vi "Interpolation Color.vi"(9 "Interpolation Value":dbl, 10 "Input Color2":u32(colorbox), 11 "Input Color1":u32(colorbox)) -> (3 "Output Color":u32(colorbox))   [LabVIEW 2020, in "3D Plot.lvclass"]
uses:
  <vilib>/Math Plots/3D Math Plots/3D Plot/3D Plot/3D Plot.lvclass
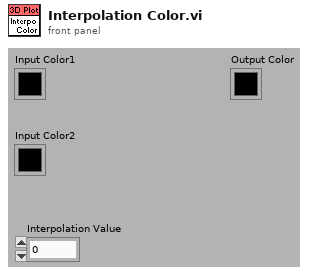
[diagram p1: front panel]
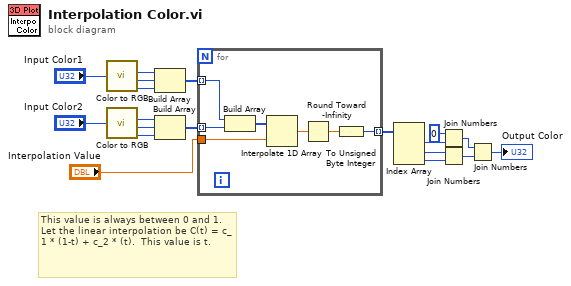
[diagram p0: block diagram]
diagram:
  # "This value is always between 0 and 1.  Let the linear interpolation be C(t) = c_1 * (1-t) + c_2 * (t).  This value is t."
  n1 = call <vilib>:"Color to RGB.vi"("Color"="Input Color1") -> ("R"=w1:u8, "G"=w2:u8, "B"=w3:u8)  [unwired: 1 out]
  n2 = call <vilib>:"Color to RGB.vi"("Color"="Input Color2") -> ("R"=w6:u8, "G"=w5:u8, "B"=w4:u8)  [unwired: 1 out]
  n3 = Build Array(w1, w2, w3) -> (w18:u8[])
  n4 = Build Array(w6, w5, w4) -> (w17:u8[])
  n5 = for {
    tunnel: w18 -> [w26] mode=indexing
    tunnel: w17 -> [w25] mode=indexing
    tunnel: "Interpolation Value" -> [w23]
    tunnel: [w20] -> w16 mode=indexing
    n6 = Build Array(w26, w25) -> (w24:u8[])
    n7 = Interpolate 1D Array(1:w23, 2:w24) -> (0:w22:dbl)
    n8 = Round Toward -Infinity(1:w22) -> (0:w21:dbl)
    n9 = To Unsigned Byte Integer(number=w21) -> (unsigned 8bit integer=w20:u8)
  }
  n10 = Index Array(array=w16) -> (element #1=w12:u8, element #2=w11:u8, element #3=w10:u8)  [unwired: 3 in]
  n11 = Join Numbers(hi=u8 0, lo=w12) -> ((hi.lo)=w14:u16)
  n12 = Join Numbers(hi=w11, lo=w10) -> ((hi.lo)=w15:u16)
  n13 = Join Numbers(hi=w14, lo=w15) -> ((hi.lo)=→"Output Color":u32)
